vi "keccak.ip.control.wrapper.vi"() -> ()   [LabVIEW 2021]
uses:
  <vilib>/Platform/TimedLoop/XDataNode/timing_clust.ctl
  <vilib>/Platform/TimedLoop/XDataNode/nitl_modes.ctl
  <vilib>/Platform/TimedLoop/XDataNode/wakeup.ctl
  <vilib>/rvi/Emulation/niFpgaSctlEmulationGetInTimedLoop.vi
  <vilib>/rvi/Emulation/niFpgaEmulationReportErrorSimple.vi
  <vilib>/rvi/Emulation/niFpgaGetClockAttributes.vi
  <vilib>/rvi/Emulation/niFpgaCriticalErrorInLSC.vi
  <vilib>/rvi/interface/RandomDataEmulation/niFpgaRandomDataHandleErrors.vi
  <vilib>/platform/TimedLoop/XDataNode/XDataNode.xnode
  <vilib>/rvi/DataTransferAndStorage/Container/XNode/niFpgaContainer.xnode
  <vilib>/rvi/interface/RandomDataEmulation/nirviRandomDataFpgaReadWriteTemplate.vi
  <vilib>/Platform/TimedLoop/XDataNode/XDNodeRunTimeDep.lvlib
panel:
  in  "Reset":bool
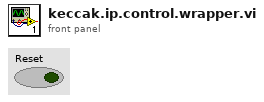
[diagram p1: front panel]
types:
  T1 = typedef "XDNodeRunTimeDep.lvlib/timing_clust.ctl" = cluster{"Expected End [f-1]":u64, "Actual End [f-1]":u64, "Finished Late? [f-1]":bool, "Expected End [i-1]":u64, "Actual End [i-1]":u64, "Finished Late? [i-1]":bool, "Expected Start [i]":u64, "Actual Start [i]":u64, "Expected Start [f]":u64, "Actual Start [f]":u64, "Source Name":string, "Structure Name":string, "Period":i64, "Deadline":i64, "Offset":i64, "Start":i64, "Priority":i32, "Timeout":i32, "Mode":T2, "Wakeup Reason":T3, "Error":errorcluster, "Source Type":string, "Secondary Source Type":string, "Global End Time":u64, "Global Start Time":u64, "Frame Duration":u64, "Iteration Duration":u64, "Assigned CPU":i32, "I/O Scan Engine Mode":u32}
  T2 = typedef "XDNodeRunTimeDep.lvlib/nitl_modes.ctl" = enum32{"No Change", "Process missed periods, maintain original phase", "Discard missed periods, maintain original phase", "Process missed periods, ignore original phase", "Discard missed periods, ignore original phase"}
  T3 = typedef "XDNodeRunTimeDep.lvlib/wakeup.ctl" = enum32{"Normal", "Aborted", "Asynchronous wakeup", "Timing source error", "Timed loop error", "Timeout"}
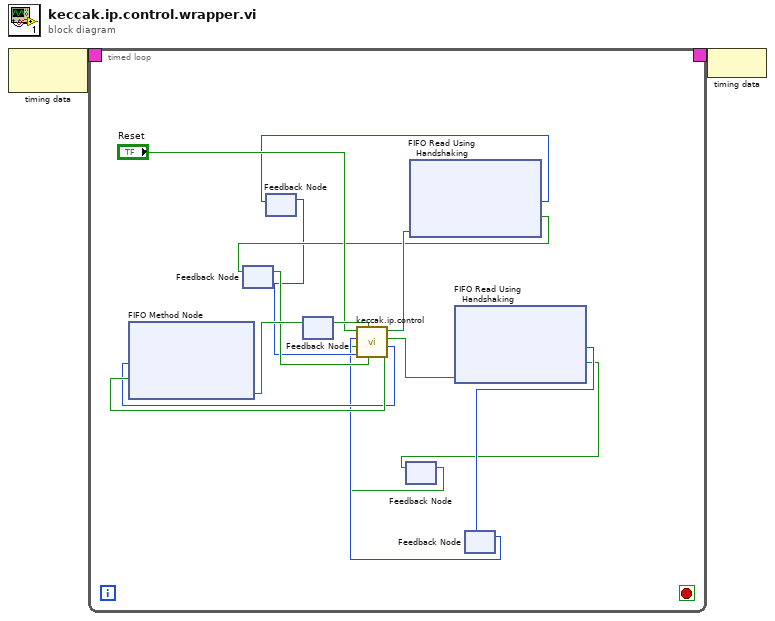
[diagram p0: block diagram]
diagram:
  n1 = node-c288() -> (w2:T1)  [unwired: 1 in]
  n2 = timed-loop {
    timing: w2 -> [_]
    timing-out: [_] -> w1
    stop <- _ stop-if-true
    n3 = feedback #1() -> (w9:bool)  [unwired: 1 in]
    n4 = feedback #2() -> (w7:u64)  [unwired: 1 in]
    n5 = feedback #3() -> (w14:bool)  [unwired: 1 in]
    n6 = feedback #4() -> (w3:bool)  [unwired: 1 in]
    n7 = feedback #5() -> (w5:u64)  [unwired: 1 in]
    n8 = call "keccak.ip.control.vi"("HT_DATA.Valid"=w9, "TH_RESULTS.Ready"=w14, "HT_DATA.Data"=w7, "HT_PARMS.Valid"=w3, "HT_PARMS.Data"=w5, "Reset"="Reset") -> ("TH_RESULTS.Valid"=w17:bool, "TH_RESULTS.Data"=w16:u64, "Read.HT_PARMS"=w13:bool, "Read.HT_DATA"=w12:bool)  [unwired: 2 in]
    n9 = xnode ("FIFO Method Node")("Element"=w16, "Input Valid"=w17) -> ("Ready for Input"=w15:bool)  [unwired: 1 in, 1 out]
    n10 = feedback-in #3(w15) -> ()
    n11 = xnode ("FIFO Read Using Handshaking")("Ready for Output"=w12) -> ("Element"=w8:u64, "Output Valid"=w10:bool)  [unwired: 1 in, 1 out]
    n12 = feedback-in #1(w10) -> ()
    n13 = feedback-in #2(w8) -> ()
    n14 = xnode ("FIFO Read Using Handshaking")("Ready for Output"=w13) -> ("Element"=w6:u64, "Output Valid"=w4:bool)  [unwired: 1 in, 1 out]
    n15 = feedback-in #4(w4) -> ()
    n16 = feedback-in #5(w6) -> ()
  }
  n17 = node-c288(w1) -> ()
